vi "Dynamic VIs.vi"   [LabVIEW 2020, in "Stream-TCP.lvlib" / "TCP Server.lvclass"]
uses:
  TCP Server/TCP Server.lvclass
  TCP Server/Server Loop Async.vi
  TCP Server/Close All Clients.vi
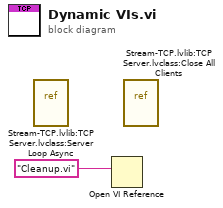
[diagram p0: block diagram]
diagram:
  n1 = vi-ref "Stream-TCP.lvlib:TCP Server.lvclass:Server Loop Async.vi"() -> ()  [unwired: 1 out]
  n2 = Open VI Reference(vi path="Cleanup.vi") -> ()  [unwired: 5 in, 2 out]
  n3 = vi-ref "Stream-TCP.lvlib:TCP Server.lvclass:Close All Clients.vi"() -> ()  [unwired: 1 out]
